vi "Obtain Queue.vi"(8 "Error In":errorcluster) -> (0 "Error Out":errorcluster, 3 "Queue out":refnum<queue>)   [LabVIEW 2019, in "IDEX.lvlib"]
uses:
  IDEX.lvlib
  Queues/Message Cluster.ctl
  Queues/Queues.lvlib
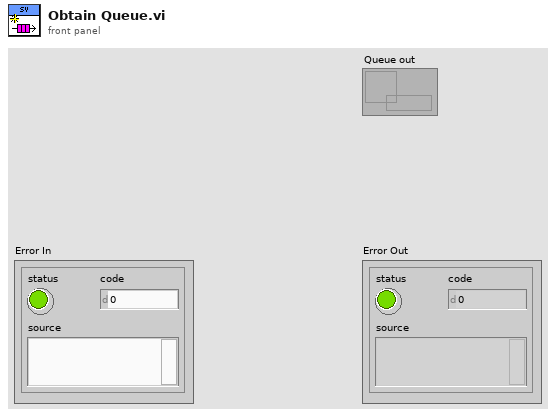
[diagram p1: front panel]
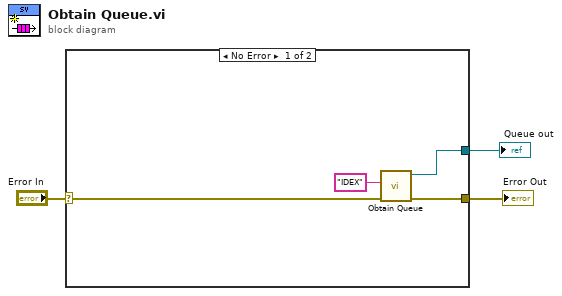
[diagram p0: block diagram]
diagram:
  n1 = case shown="No Error" "Error In" {
    selector: "Error In" -> [w6 w8]
    tunnel: [w5 w8] -> w3
    tunnel: [w7 _] -> w1
    frame No Error {
      n2 = call "Obtain Queue.vi"("Error In"=w6, "Queue Name"="IDEX" ("name (unnamed)")) -> ("Error Out"=w5:errorcluster, "queue out"=w7:refnum<queue>)  [unwired: 8 in]
    }
    frame Error {
    }
  }
  "Error Out" <- w3
  "Queue out" <- w1
